vi "populate, show and serialize.vi"() -> ()   [LabVIEW 2018]
uses:
  _Serializable Base Object/_ISerializable.lvclass
  Implementations/Component-A.lvclass
  U:/modules/labview-orm/_Serializable Base Object/_ISerializable.lvclass
  U:/modules/labview-orm/demo/Component.lvclass
  Implementations/Product-A.lvclass
  U:/modules/labview-orm/demo/Product.lvclass
  ORM/LV-ORM.lvclass
  ORM Scripter/ORM Scripter.lvclass
panel:
  out "all products":refnum<class "_ISerializable.lvclass">[](array[class])
  out "all components":refnum<class "_ISerializable.lvclass">[](array[class])
  out "components":string[][](array[string])
  out "products":string[][](array[string])
  out "xml string":string
  out "error out 2":errorcluster
  out "error out":errorcluster
  out "create script 3":string
  out "create script":string
  # "CREATE TYPE mood AS ENUM    ->\n('sad', 'ok', 'happy');"
  # "CREATE TYPE complex AS (    ->\n    r       double precision,\n    i       double precision\n);"
  # "TIMESTAMPZ\n(with timezone)"
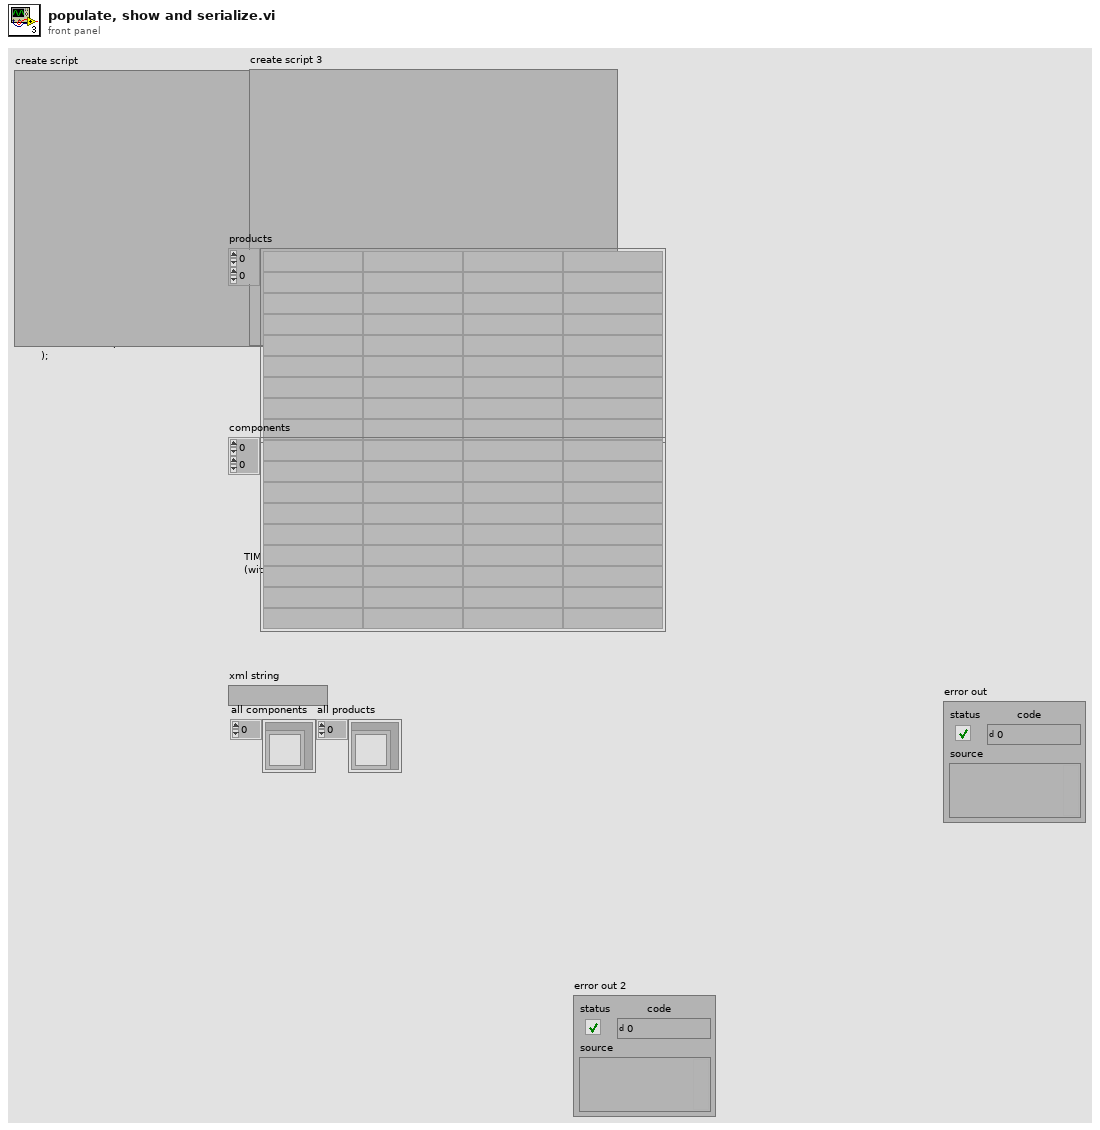
[diagram p1: front panel]
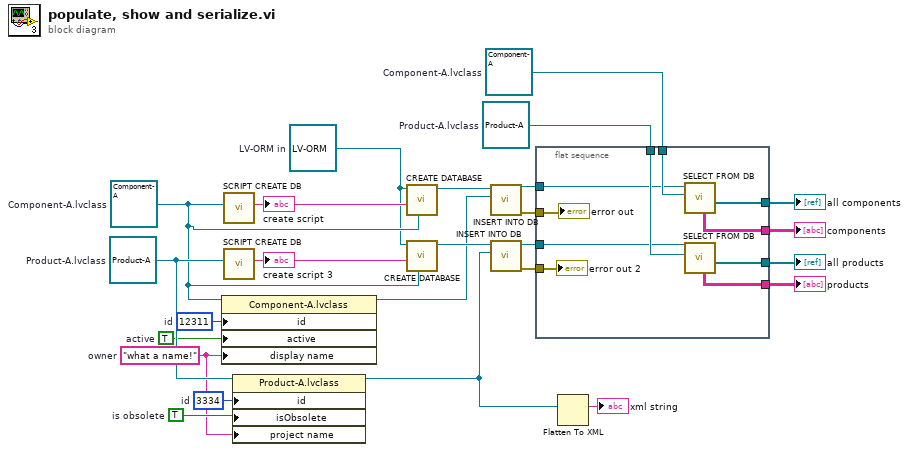
[diagram p0: block diagram]
diagram:
  w7 = refnum<class "LV-ORM.lvclass"> refnum  # LV-ORM in
  w12 = refnum<class "Product-A.lvclass"> refnum  # Product-A.lvclass
  w11 = refnum<class "Component-A.lvclass"> refnum  # Component-A.lvclass
  w17 = TRUE  # is obsolete
  w18 = 3334  # id
  w16 = "what a name!"  # owner
  w19 = 12311  # id
  w20 = TRUE  # active
  w21 = refnum<class "Product-A.lvclass"> refnum  # Product-A.lvclass
  w8 = refnum<class "Component-A.lvclass"> refnum  # Component-A.lvclass
  n1 = property class="Component-A.lvclass"(reference=w8, "id"=w19, "active"=w20, "display name"=w16) -> (reference out=w15:refnum<class "Component-A.lvclass">)  [unwired: 1 in, 1 out]
  n2 = call "SCRIPT CREATE DB.vi"("class"=w8) -> ("create script"=w25:string)  [unwired: 8 in, 2 out]
  "create script" <- w25
  n3 = call "SCRIPT CREATE DB.vi"("class"=w21) -> ("create script"=w24:string)  [unwired: 8 in, 2 out]
  "create script 3" <- w24
  n4 = property class="Product-A.lvclass"(reference=w21, "id"=w18, "isObsolete"=w17, "project name"=w16) -> (reference out=w6:refnum<class "Product-A.lvclass">)  [unwired: 1 in, 1 out]
  n5 = call "CREATE DATABASE.vi"("object"=w8, "create script 2"=w25, "LV-ORM in"=w7) -> ("LV-ORM out"=w23:refnum<class "LV-ORM.lvclass">)  [unwired: 8 in]
  n6 = call "CREATE DATABASE.vi"("object"=w8, "create script 2"=w24, "LV-ORM in"=w7) -> ("LV-ORM out"=w22:refnum<class "LV-ORM.lvclass">)  [unwired: 8 in]
  n7 = call "INSERT INTO DB.vi"("object"=w15, "orm in"=w23) -> ("error out"=w14:errorcluster, "orm out"=w10:refnum<class "LV-ORM.lvclass">)  [unwired: 8 in]
  n8 = call "INSERT INTO DB.vi"("object"=w6, "orm in"=w22) -> ("error out"=w13:errorcluster, "orm out"=w9:refnum<class "LV-ORM.lvclass">)  [unwired: 8 in]
  n9 = flat-sequence {
    tunnel: w14 -> [w35]
    tunnel: w13 -> [w34]
    tunnel: w12 -> [w33]
    tunnel: w11 -> [w32]
    tunnel: w10 -> [w31]
    tunnel: w9 -> [w30]
    tunnel: [w29] -> w2
    tunnel: [w28] -> w1
    tunnel: [w27] -> w4
    tunnel: [w26] -> w3
    frame #0 {
      n10 = call "SELECT FROM DB.vi"("object"=w32, "orm in"=w31) -> ("all obj"=w29:refnum<class "_ISerializable.lvclass">[], "data"=w26:string[][])  [unwired: 5 in, 3 out]
      n11 = call "SELECT FROM DB.vi"("object"=w33, "orm in"=w30) -> ("all obj"=w28:refnum<class "_ISerializable.lvclass">[], "data"=w27:string[][])  [unwired: 5 in, 3 out]
      "error out" <- w35
      "error out 2" <- w34
    }
  }
  n12 = Flatten To XML(anything=w6) -> (xml string=→"xml string":string)
  "products" <- w4
  "components" <- w3
  "all components" <- w2
  "all products" <- w1
